vi "Set Count Convert Wavelength.vi"(11 "wavelength":sgl) -> (3 "function return":u32)   [LabVIEW 2018, in "AndorSDK.lvlib"]
doc: "EXPNETTYPE unsigned int WINAPI SetCountConvertWavelength(float wavelength);"
uses:
  AndorSDK.lvlib
  ATMCD32D.dll
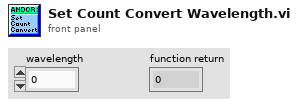
[diagram p1: front panel]
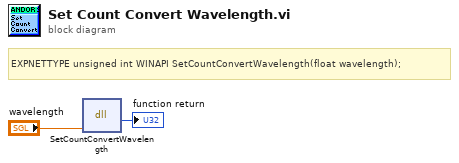
[diagram p0: block diagram]
diagram:
  # "EXPNETTYPE unsigned int WINAPI SetCountConvertWavelength(float wavelength);"
  n1 = dll-call lib="PTH2babs E\nPersönliches02 - Arbeit03-HiwijobsLabviewCodelibANDOR\tAndor SDK\nATMCD32D.*" fn="SetCountConvertWavelength"("wavelength"="wavelength") -> (→"function return":u32)  [unwired: 4 in, 2 out]
